vi "Test Threshold Estimation.vi"() -> ()   [LabVIEW 2020]
uses:
  ABR3-Threshold Estimation Parameters.ctl
panel:
  in  "Threshold Estimation":T1={"Tmin (ms)"=0.0, "Tmax (ms)"=8.5, "CC criterion"=0.35, "adjR2 criterion"=0.7}
  in  "Path":path=path "D:/Data/ABR exemplars/ABR-102-1"
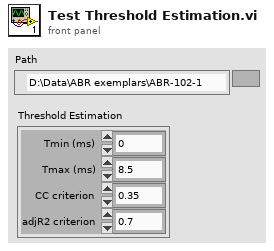
[diagram p1: front panel]
types:
  T1 = typedef "ABR3-Threshold Estimation Parameters.ctl" = cluster{"Tmin (ms)":dbl, "Tmax (ms)":dbl, "CC criterion":dbl, "adjR2 criterion":dbl}
  T2 = typedef "ABR-Analysis State.ctl" = cluster{"dt (us)":dbl, "Neural":dbl[][], "CM":dbl[][], "Metrics":dbl[][], "Level":dbl[], "Avgs":i32[], "Attempts":i32[], "Aborted":bool, "threshold":dbl, "Lnominal":dbl[], "tone":bool, "work":bool, "ThrResult":T3, "ITI":dbl}
  T3 = typedef "ABR3-Threshold Estimation Result.ctl" = enum16{"None", "Power", "Sigmoid", "Power (noisy)", "Suprathreshold", "Invalid"}
  T4 = typedef "ABR3-Threshold Estimation Work.ctl" = cluster{"Threshold":dbl, "Criterion":dbl, "graphs":cluster{"X":dbl[], "Y":dbl[]}[], "Power2":string, "Sigmoid":string, "Result":T3}
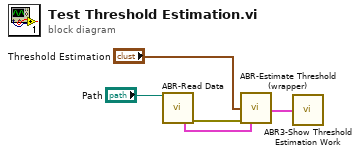
[diagram p0: block diagram]
diagram:
  n1 = call "ABR-Read Data.vi"("Path"="Path") -> ("Analysis"=w2:T2, "error out"=w3:errorcluster)  [unwired: 9 in, 4 out]
  n2 = call "ABR-Estimate Threshold (wrapper).vi"("Threshold Estimation"="Threshold Estimation", "error in (no error)"=w3, "Analysis (in)"=w2) -> ("Work"=w1:T4)  [unwired: 10 in, 2 out]
  n3 = call "ABR3-Show Threshold Estimation Work.vi"("work"=w1) -> ()  [unwired: 15 in]
